vi "Modbus Master Example.vi"() -> ()   [LabVIEW 2015, in "Modbus Library.lvlib"]
doc: "An example of the modbus master functionality."
uses:
  Modbus Library.lvlib
  API/Master/Modbus Master.lvclass
  Master Function Definition/Read Device ID code.ctl
  API/Wrapper/Create TCP Master.vi
  API/Wrapper/API Main.lvlib
  Data Model/Device Data Model.lvclass
panel:
  in  "Stop Button":bool
  in  "Port":u16=502
  in  "Set Holding Registers":bool
  in  "Set Coils":bool
  in  "Fetch Discrete Inputs":bool
  in  "Fetch Input Registers":bool
  in  "Fetch Basic Objects":bool
  out "Basic Objects":string[](array[string])
  out "Status":string
  in  "Disconnect":bool
  in  "Connect":bool
  in  "Holding Registers":u16[](array[numeric])=[0, 0, 0, 0, 0, 0, 0, 0]
  out "Input Registers":u16[](array[numeric])
  in  "Coils":bool[](array[boolean])=[FALSE, FALSE, FALSE, FALSE, FALSE, FALSE, FALSE, FALSE]
  out "Discrete Inputs":bool[](array[boolean])
  in  "Slave Address":string="localhost"
  # "Coils are the boolean outputs of a modbus device. This example allows you to set the first 8 outputs."
  # "Holding Registers are the integer outputs of a modbus device. This example allows you to set the first 8 outputs."
  # "Modbus devices can also store objects in their memory, which are variable length strings. This example requests the basic level of objects."
  # "Discrete inputs are the boolean inputs of a modbus device. This example allows you to read the first 8 inputs."
  # "Input Registers are the integer inputs of a modbus device. This example allows you to read the first 8 inputs."
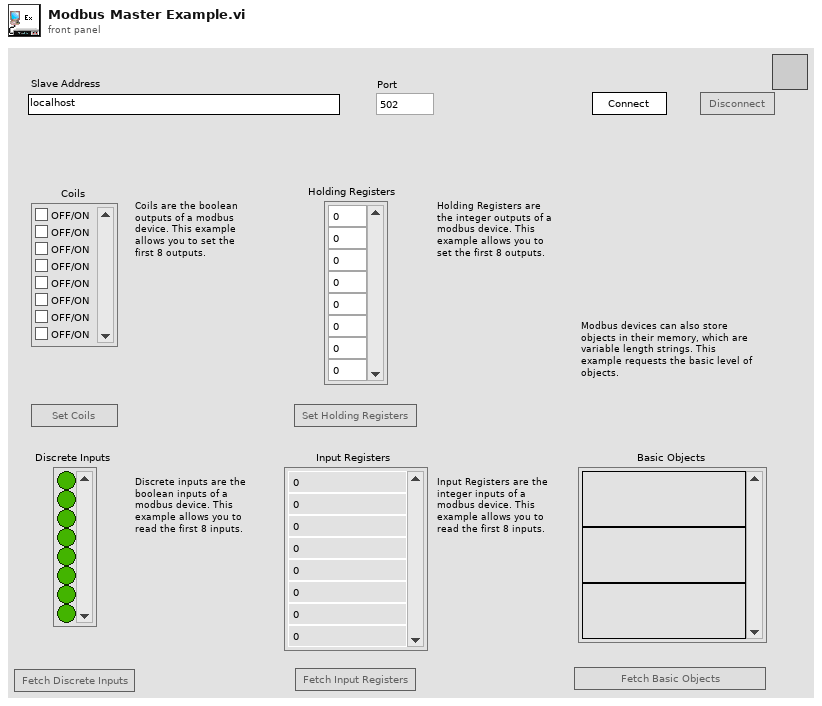
[diagram p1: front panel]
types:
  T1 = enum8{"Enabled", "Disabled", "Disabled and Grayed Out"}
  T2 = typedef "Modbus Library.lvlib/Device Data Model.lvclass/Read Device ID code.ctl" = enum8{"Read Basic", "Read Regular", "Read Extended", "Read Specific"}
  T3 = typedef "Modbus Library.lvlib/Device Data Model.lvclass/Identification Parameters.ctl" = cluster{"Object ID":u8, "Value":string}
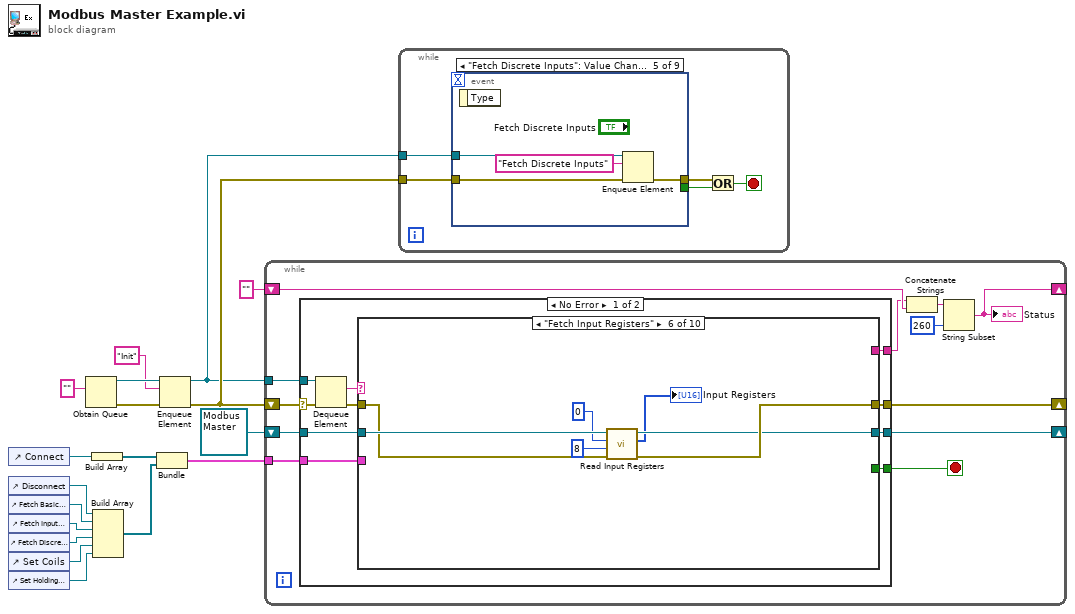
[diagram p0: block diagram]
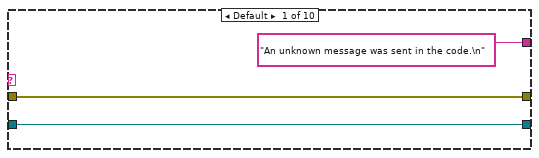
[diagram p2: hidden frame]
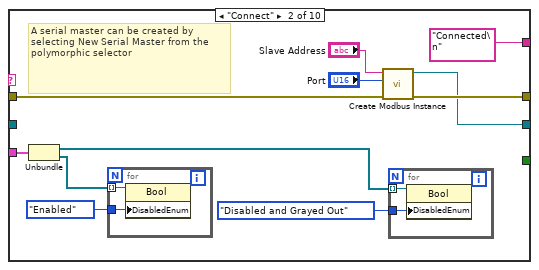
[diagram p3: hidden frame]
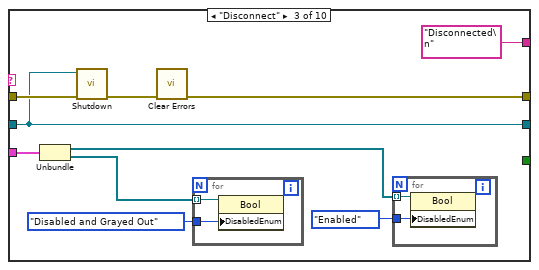
[diagram p4: hidden frame]
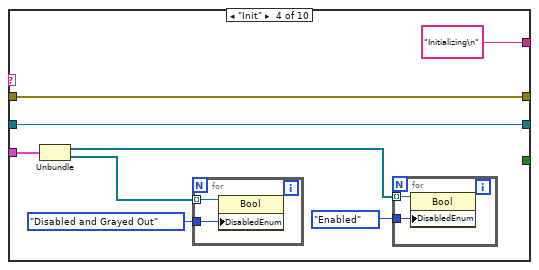
[diagram p5: hidden frame]
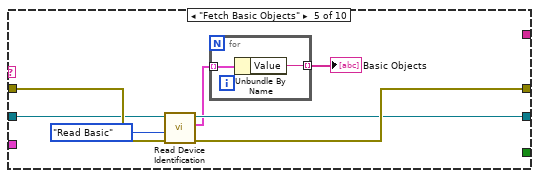
[diagram p6: hidden frame]
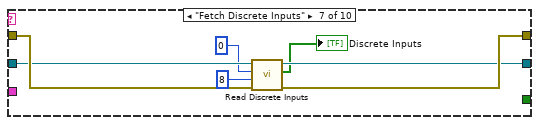
[diagram p7: hidden frame]
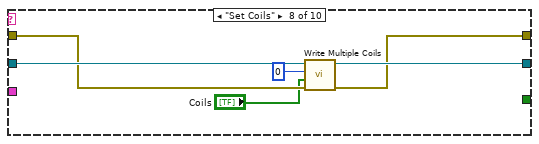
[diagram p8: hidden frame]
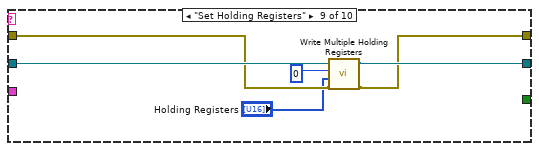
[diagram p9: hidden frame]
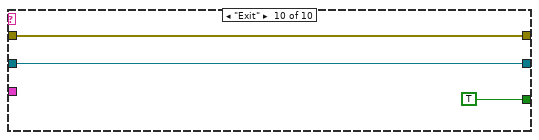
[diagram p10: hidden frame]
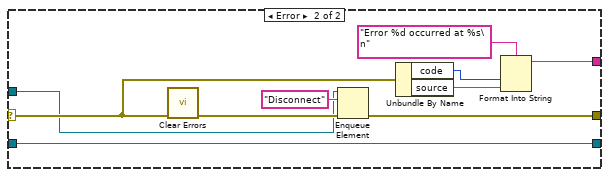
[diagram p11: hidden frame]
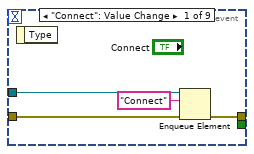
[diagram p12: hidden frame]
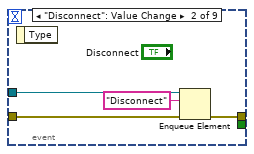
[diagram p13: hidden frame]
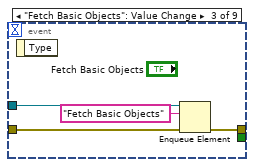
[diagram p14: hidden frame]
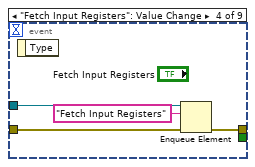
[diagram p15: hidden frame]
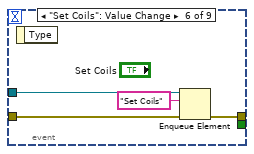
[diagram p16: hidden frame]
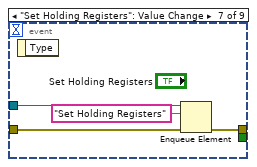
[diagram p17: hidden frame]
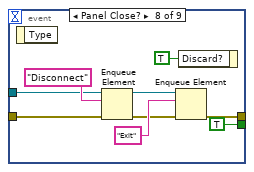
[diagram p18: hidden frame]
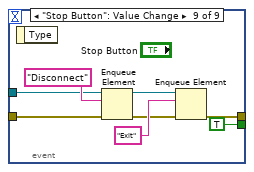
[diagram p19: hidden frame]
diagram:
  n1 = control-ref of="Connect"() -> (w9:refnum<vi>)
  n2 = control-ref of="Disconnect"() -> (w15:refnum<vi>)
  n3 = control-ref of="Fetch Basic Objects"() -> (w14:refnum<vi>)
  n4 = control-ref of="Fetch Input Registers"() -> (w13:refnum<vi>)
  n5 = control-ref of="Fetch Discrete Inputs"() -> (w12:refnum<vi>)
  n6 = control-ref of="Set Coils"() -> (w11:refnum<vi>)
  n7 = control-ref of="Set Holding Registers"() -> (w10:refnum<vi>)
  n8 = Obtain Queue(element data type="") -> (queue out=w4:refnum<queue>, error out=w18:errorcluster)  [unwired: 4 in, 1 out]
  n9 = Build Array(w9) -> (w6:refnum<vi>[])
  n10 = Build Array(w15, w14, w13, w12, w11, w10) -> (w8:refnum<vi>[])
  n11 = Bundle(w6, w8) -> (w7:cluster{refnum<vi>[], refnum<vi>[]})  [unwired: 1 in]
  n12 = Enqueue Element(queue=w4, element="Init", error in (no error)=w18) -> (queue out=w3:refnum<queue>, error out=w5:errorcluster)  [unwired: 1 in, 1 out]
  n13 = while {
    shift-right: [w22] -> _
    shift-left: refnum<class "Modbus Master.lvclass"> refnum ("Modbus Master") -> [w21]
    tunnel: w3 -> [w30]
    shift-right: [w28] -> _
    shift-left: w5 -> [w29]
    shift-right: [w27] -> _
    shift-left: "" ("Status") -> [w24]
    tunnel: w7 -> [w19]
    stop <- w20 stop-if-true
    n14 = case shown="No Error" w29 {
      selector: w29 -> [w39 w130]
      tunnel: w30 -> [w40 w124]
      tunnel: [w36 w131] -> w28
      tunnel: [w33 w127] -> w23
      tunnel: [w35 w123] -> w22
      tunnel: w21 -> [w34 w123]
      tunnel: [w32 _] -> w20
      tunnel: w19 -> [w31 _]
      frame No Error {
        n15 = Dequeue Element(queue=w40, error in (no error)=w39) -> (element=w37:string, error out=w38:errorcluster)  [unwired: 1 in, 2 out]
        n16 = case shown="\"Fetch Input Registers\"" w37 {
          tunnel: w38 -> [w43 w53 w68 w80 w91 w97 w107 w110 w116 w122]
          tunnel: [w43 w52 w64 w80 w90 w100 w106 w111 w117 w122] -> w36
          tunnel: [w42 w51 w66 w79 w88 w99 w104 w112 w118 w121] -> w35
          tunnel: w34 -> [w42 _ w66 w79 w89 w98 w105 w113 w119 w121]
          tunnel: ["An unknown message was sent in the code.\n" "Connected\n" "Disconnected\n" "Initializing\n" _ _ _ _ _ _] -> w33
          tunnel: [_ _ _ _ _ _ _ _ _ TRUE] -> w32
          tunnel: w31 -> [_ w49 w63 w77 _ _ _ _ _ _]
          frame Default {
          }
          frame "Connect" {
            # "A serial master can be created by selecting New Serial Master from the polymorphic selector"
            n17 = Unbundle(w49) -> (w47:refnum<vi>[], w48:refnum<vi>[])
            n18 = for {
              tunnel: w48 -> [w56] mode=indexing
              tunnel: T1."Enabled" ("Disabled") -> [w55]
              n19 = property class="Bool"(reference=w56, "DisabledEnum"=w55) -> ()  [unwired: 1 in, 2 out]
            }
            n20 = call-poly "Create Modbus Instance.vi"("error in"=w53, "port (502)"="Port", "address"="Slave Address") -> ("error out"=w52:errorcluster, "TCP master instance"=w51:refnum<class "Modbus Master.lvclass">)  [unwired: 7 in]
            n21 = for {
              tunnel: w47 -> [w58] mode=indexing
              tunnel: T1."Disabled and Grayed Out" ("Disabled") -> [w57]
              n22 = property class="Bool"(reference=w58, "DisabledEnum"=w57) -> ()  [unwired: 1 in, 2 out]
            }
          }
          frame "Disconnect" {
            n23 = Unbundle(w63) -> (w61:refnum<vi>[], w62:refnum<vi>[])
            n24 = call-dynamic "Shutdown.vi"("error in"=w68, "Modbus master in"=w66) -> ("error out"=w67:errorcluster)  [unwired: 9 in]
            n25 = call <vilib>:"Clear Errors.vi"("error in (no error)"=w67) -> ("error out"=w64:errorcluster)  [unwired: 5 in, 1 out]
            n26 = for {
              tunnel: w62 -> [w72] mode=indexing
              tunnel: T1."Disabled and Grayed Out" ("Disabled") -> [w71]
              n27 = property class="Bool"(reference=w72, "DisabledEnum"=w71) -> ()  [unwired: 1 in, 2 out]
            }
            n28 = for {
              tunnel: w61 -> [w70] mode=indexing
              tunnel: T1."Enabled" ("Disabled") -> [w69]
              n29 = property class="Bool"(reference=w70, "DisabledEnum"=w69) -> ()  [unwired: 1 in, 2 out]
            }
          }
          frame "Init" {
            n30 = Unbundle(w77) -> (w75:refnum<vi>[], w76:refnum<vi>[])
            n31 = for {
              tunnel: w76 -> [w84] mode=indexing
              tunnel: T1."Disabled and Grayed Out" ("Disabled") -> [w83]
              n32 = property class="Bool"(reference=w84, "DisabledEnum"=w83) -> ()  [unwired: 1 in, 2 out]
            }
            n33 = for {
              tunnel: w75 -> [w82] mode=indexing
              tunnel: T1."Enabled" ("Disabled") -> [w81]
              n34 = property class="Bool"(reference=w82, "DisabledEnum"=w81) -> ()  [unwired: 1 in, 2 out]
            }
          }
          frame "Fetch Basic Objects" {
            n35 = call-dynamic "Read Device Identification.vi"("error in"=w91, "read device ID code"=Read_Device_ID_code."Read Basic" ("Read Device ID code"), "Modbus master in"=w89) -> ("error out"=w90:errorcluster, "objects"=w86:T3[], "Modbus master out"=w88:refnum<class "Modbus Master.lvclass">)  [unwired: 6 in]
            n36 = for {
              tunnel: w86 -> [w93] mode=indexing
              tunnel: [w92] -> w85 mode=indexing
              n37 = Unbundle By Name(w93) -> ("Value"=w92:string)
            }
            "Basic Objects" <- w85
          }
          frame "Fetch Input Registers" {
            n38 = call-dynamic "Read Input Registers.vi"("error in"=w97, "number of inputs"=u16 8 ("number of registers"), "starting address"=u16 0, "Modbus master in"=w98) -> ("error out"=w100:errorcluster, "register values"=→"Input Registers":u16[], "Modbus master out"=w99:refnum<class "Modbus Master.lvclass">)  [unwired: 5 in]
          }
          frame "Fetch Discrete Inputs" {
            n39 = call-dynamic "Read Discrete Inputs.vi"("error in"=w107, "number of inputs"=u16 8, "starting address"=u16 0, "Modbus master in"=w105) -> ("error out"=w106:errorcluster, "discrete inputs"=→"Discrete Inputs":bool[], "Modbus master out"=w104:refnum<class "Modbus Master.lvclass">)  [unwired: 5 in]
          }
          frame "Set Coils" {
            n40 = call-dynamic "Write Multiple Coils.vi"("error in"=w110, "coils to write"="Coils", "starting address"=u16 0, "Modbus master in"=w113) -> ("error out"=w111:errorcluster, "Modbus master out"=w112:refnum<class "Modbus Master.lvclass">)  [unwired: 6 in]
          }
          frame "Set Holding Registers" {
            n41 = call-dynamic "Write Multiple Holding Registers.vi"("error in"=w116, "registers to write"="Holding Registers", "starting address"=u16 0, "Modbus master in"=w119) -> ("error out"=w117:errorcluster, "Modbus master out"=w118:refnum<class "Modbus Master.lvclass">)  [unwired: 6 in]
          }
          frame "Exit" {
          }
        }
      }
      frame Error {
        n42 = call <vilib>:"Clear Errors.vi"("error in (no error)"=w130) -> ("error out"=w132:errorcluster)  [unwired: 5 in, 1 out]
        n43 = Enqueue Element(queue=w124, element="Disconnect", error in (no error)=w132) -> (error out=w131:errorcluster)  [unwired: 1 in, 2 out]
        n44 = Unbundle By Name(w130) -> ("code"=w129:i32, "source"=w128:string)
        n45 = Format Into String(format string="Error %d occurred at %s\n", w129, w128) -> (resulting string=w127:string)  [unwired: 2 in, 1 out]
      }
    }
    n46 = Concatenate Strings(w23, w24) -> (w25:string)
    n47 = String Subset(string=w25, length (rest)=260 ("length (rest)")) -> (substring=w27:string)  [unwired: 1 in]
    "Status" <- w27
  }
  n48 = while {
    tunnel: w5 -> [w137]
    tunnel: w3 -> [w136]
    stop <- w133 stop-if-true
    n49 = event shown="[4] \"Fetch Discrete Inputs\": Value Change" {
      selector: _ -> [_ _ _ _ _ _ _ _ _]
      dyn-events: _ -> [_ _ _ _ _ _ _ _ _]
      timeout: _ -> [_ _ _ _ _ _ _ _ _]
      tunnel: w137 -> [w141 w145 w149 w153 w157 w161 w165 w171 w180]
      tunnel: [w140 w144 w148 w152 w156 w160 w164 w166 w175] -> w135
      tunnel: w136 -> [w139 w143 w147 w151 w155 w159 w163 w168 w177]
      tunnel: [_ _ _ _ _ _ _ TRUE ("Discard?") TRUE ("Discard?")] -> w134
      event "Connect": Value Change {
        n50 = event-data() -> ()  [unwired: 1 in, 1 out]
        n51 = Enqueue Element(queue=w139, element="Connect", error in (no error)=w141) -> (error out=w140:errorcluster)  [unwired: 1 in, 2 out]
      }
      event "Disconnect": Value Change {
        n52 = event-data() -> ()  [unwired: 1 in, 1 out]
        n53 = Enqueue Element(queue=w143, element="Disconnect", error in (no error)=w145) -> (error out=w144:errorcluster)  [unwired: 1 in, 2 out]
      }
      event "Fetch Basic Objects": Value Change {
        n54 = event-data() -> ()  [unwired: 1 in, 1 out]
        n55 = Enqueue Element(queue=w147, element="Fetch Basic Objects", error in (no error)=w149) -> (error out=w148:errorcluster)  [unwired: 1 in, 2 out]
      }
      event "Fetch Input Registers": Value Change {
        n56 = event-data() -> ()  [unwired: 1 in, 1 out]
        n57 = Enqueue Element(queue=w151, element="Fetch Input Registers", error in (no error)=w153) -> (error out=w152:errorcluster)  [unwired: 1 in, 2 out]
      }
      event "Fetch Discrete Inputs": Value Change {
        n58 = event-data() -> ()  [unwired: 1 in, 1 out]
        n59 = Enqueue Element(queue=w155, element="Fetch Discrete Inputs", error in (no error)=w157) -> (error out=w156:errorcluster)  [unwired: 1 in, 2 out]
      }
      event "Set Coils": Value Change {
        n60 = event-data() -> ()  [unwired: 1 in, 1 out]
        n61 = Enqueue Element(queue=w159, element="Set Coils", error in (no error)=w161) -> (error out=w160:errorcluster)  [unwired: 1 in, 2 out]
      }
      event "Set Holding Registers": Value Change {
        n62 = event-data() -> ()  [unwired: 1 in, 1 out]
        n63 = Enqueue Element(queue=w163, element="Set Holding Registers", error in (no error)=w165) -> (error out=w164:errorcluster)  [unwired: 1 in, 2 out]
      }
      event Panel Close? {
        n64 = event-data() -> ()  [unwired: 1 in, 1 out]
        n65 = Enqueue Element(queue=w168, element="Disconnect", error in (no error)=w171) -> (queue out=w169:refnum<queue>, error out=w167:errorcluster)  [unwired: 1 in, 1 out]
        n66 = Enqueue Element(queue=w169, element="Exit", error in (no error)=w167) -> (error out=w166:errorcluster)  [unwired: 1 in, 2 out]
        n67 = event-data("Discard?"=TRUE) -> ()  [unwired: 1 in, 1 out]
      }
      event "Stop Button": Value Change {
        n68 = event-data() -> ()  [unwired: 1 in, 1 out]
        n69 = Enqueue Element(queue=w177, element="Disconnect", error in (no error)=w180) -> (queue out=w178:refnum<queue>, error out=w176:errorcluster)  [unwired: 1 in, 1 out]
        n70 = Enqueue Element(queue=w178, element="Exit", error in (no error)=w176) -> (error out=w175:errorcluster)  [unwired: 1 in, 2 out]
      }
    }
    n71 = Or(x=w135, y=w134) -> (x .or. y?=w133:bool)
  }
